vi "Stream Line (FW7).vi"(6 "Position Mode (0: absolute)":u16(ring) items=["absolute", "relative"], 7 "Coordinates":i64[](array[numeric]), 8 "error in (no error)":errorcluster, 9 "Device Number":string, 10 "Stream Number (1)":u8=1, 11 "VISA resource name":refnum<visa-resource-name>) -> (0 "error out":errorcluster, 3 "VISA resource name out":refnum<visa-resource-name>)   [LabVIEW 2018, in "Zaber A Series.lvlib"]
doc: "Adds a line command to an open stream. The line will always start where the previous stream command leaves the device positioned. The endpoint can be specified relative to there, or in absolute coordinates. The endpoint is specified in microstep units - use the Convert Position to Device Units VI to convert from standard measurements.\n\nThis VI does not check in advance for error conditions such as streams not being supported or the stream not being open.\n\nThis VI requires that the Initialize VI has been called with the same serial port and that the specified stream is open."
uses:
  Zaber A Series.lvlib
  Private/All Commands.ctl
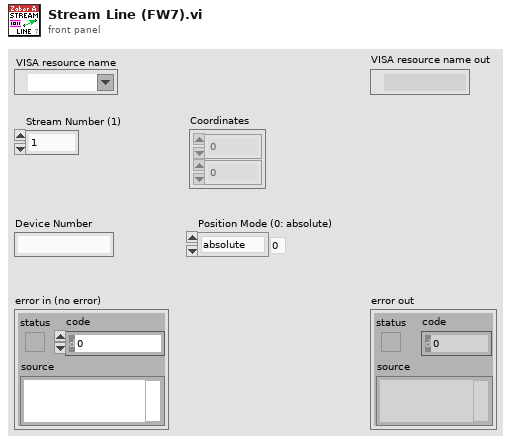
[diagram p1: front panel]
types:
  T1 = typedef "Zaber A Series.lvlib/All Commands.ctl" = string
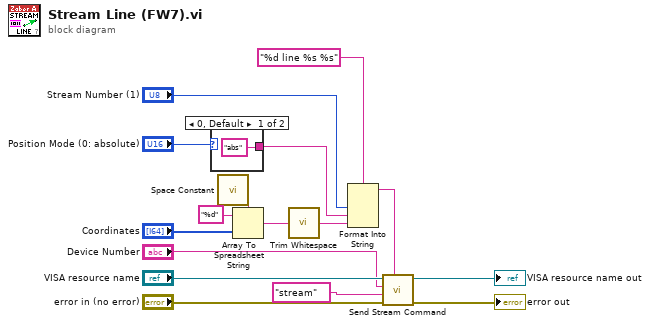
[diagram p0: block diagram]
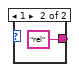
[diagram p2: hidden frame]
diagram:
  n1 = case shown="0, Default" "Position Mode (0: absolute)" {
    tunnel: ["abs" "rel"] -> w4
    frame 0, Default {
    }
    frame 1 {
    }
  }
  n2 = call <vilib>:"Space Constant.vi"() -> ("String"=w13:string)
  n3 = Array To Spreadsheet String(delimiter (Tab)=w13, array="Coordinates", 3:"%d" ("format string")) -> (spreadsheet string=w7:string)
  n4 = call <vilib>:"Trim Whitespace.vi"("string"=w7) -> ("trimmed string"=w3:string)  [unwired: 1 in]
  n5 = Format Into String(format string="%d line %s %s", "Stream Number (1)", w4, w3) -> (resulting string=w2:string)  [unwired: 2 in, 1 out]
  n6 = call "Send Stream Command.vi"("Data"=w2, "error in (no error)"="error in (no error)", "Command"=T1 "stream" ("Complete Command List"), "Device Number"="Device Number", "VISA resource name"="VISA resource name") -> ("error out"=→"error out":errorcluster, "VISA resource name out"=→"VISA resource name out":refnum<visa-resource-name>)  [unwired: 5 in]
